vi "writeBinningXML.vi"(8 "error in (no error)":errorcluster, 10 "NativeXML in":refnum<class "NativeXML.lvclass">, 11 "PixelflySettings in":refnum<class "PixelflySettings.lvclass">) -> (0 "error out":errorcluster, 2 "NativeXML out":refnum<class "NativeXML.lvclass">, 3 "PixelflySettings out":refnum<class "PixelflySettings.lvclass">)   [LabVIEW 2011, in "Tools.lvlib" / "Settings.lvlib" / "PixelflySettings.lvclass"]
uses:
  PixelflySettings.lvclass
  NativeXML/NativeXML.lvclass
  PixelflySettings.lvclass/PixelflySettings.ctl
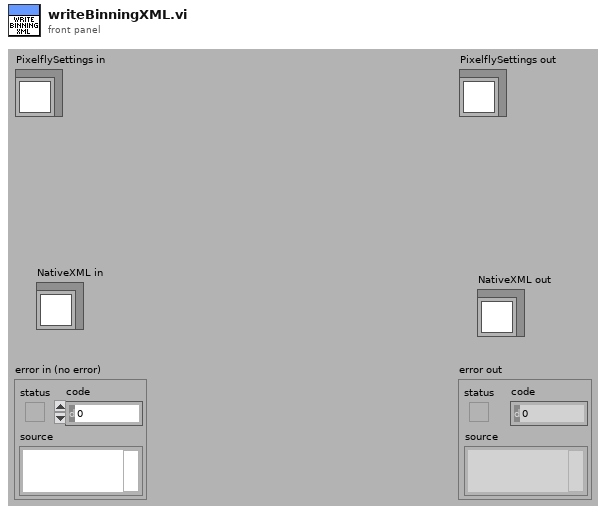
[diagram p1: front panel]
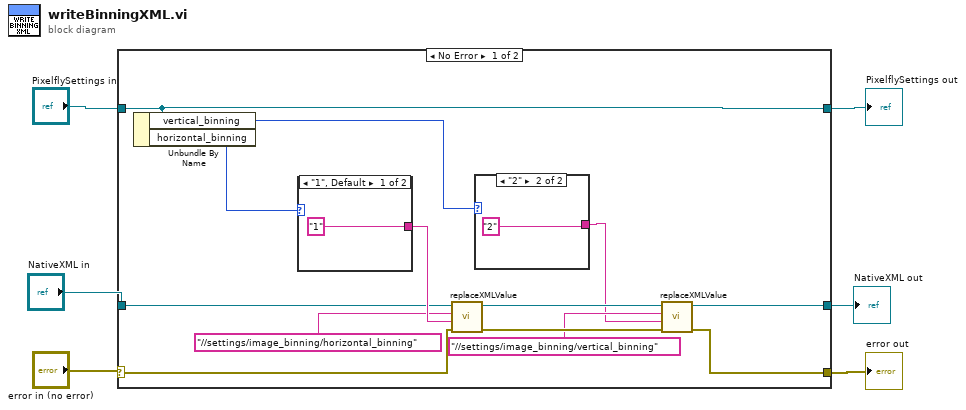
[diagram p0: block diagram]
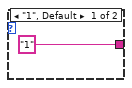
[diagram p2: hidden frame]
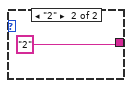
[diagram p3: hidden frame]
diagram:
  n1 = case shown="No Error" "error in (no error)" {
    selector: "error in (no error)" -> [w15 w26]
    tunnel: [w8 w26] -> w5
    tunnel: [w16 w25] -> w6
    tunnel: "PixelflySettings in" -> [w16 w25]
    tunnel: "NativeXML in" -> [w14 w24]
    tunnel: [w7 w24] -> w1
    frame No Error {
      n2 = Unbundle By Name(w16) -> ("vertical_binning"=w11:enum16{"1", "2"}, "horizontal_binning"=w19:enum16{"1", "2"})
      n3 = case shown="\"1\", Default" w19 {
        tunnel: ["1" "2"] -> w18
        frame "1", Default {
        }
        frame "2" {
        }
      }
      n4 = call "replaceXMLValue.vi"("error in (no error)"=w15, "value"=w18, "replace in"="//settings/image_binning/horizontal_binning", "NativeXML in"=w14) -> ("error out"=w12:errorcluster, "NativeXML out"=w13:refnum<class "NativeXML.lvclass">)  [unwired: 6 in]
      n5 = case shown="\"2\"" w11 {
        tunnel: ["1" "2"] -> w9
        frame "1", Default {
        }
        frame "2" {
        }
      }
      n6 = call "replaceXMLValue.vi"("error in (no error)"=w12, "value"=w9, "replace in"="//settings/image_binning/vertical_binning", "NativeXML in"=w13) -> ("error out"=w8:errorcluster, "NativeXML out"=w7:refnum<class "NativeXML.lvclass">)  [unwired: 6 in]
    }
    frame Error {
    }
  }
  "error out" <- w5
  "PixelflySettings out" <- w6
  "NativeXML out" <- w1
